vi "Run Static.vi"(7 "Tester":refnum<class "Tester.lvclass">, 8 "error in (no error)":errorcluster, 11 "Step in":refnum<class "Step.lvclass">) -> (0 "error out":errorcluster, 3 "Step out":refnum<class "Step.lvclass">)   [LabVIEW 2020, in "Tester.lvlib" / "Step.lvclass"]
uses:
  Step.lvclass
  Tester/Tester.lvclass
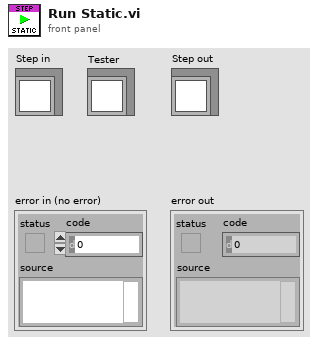
[diagram p1: front panel]
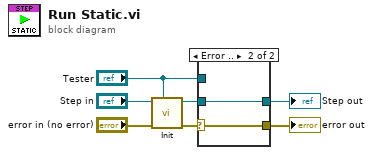
[diagram p0: block diagram]
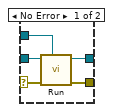
[diagram p2: hidden frame]
diagram:
  n1 = call-dynamic "Init.vi"("Tester"="Tester", "error in (no error)"="error in (no error)", "Step in"="Step in") -> ("error out"=w5:errorcluster, "Step out"=w4:refnum<class "Step.lvclass">)  [unwired: 7 in]
  n2 = case shown="Error .." w5 {
    selector: w5 -> [w11 w13]
    tunnel: w4 -> [w12 w14]
    tunnel: [w10 w14] -> w1
    tunnel: "Tester" -> [w9 _]
    tunnel: [w8 w13] -> w2
    frame No Error {
      n3 = call-dynamic "Run.vi"("Tester"=w9, "error in (no error)"=w11, "Step in"=w12) -> ("error out"=w8:errorcluster, "Step out"=w10:refnum<class "Step.lvclass">)  [unwired: 7 in]
    }
    frame Error {
    }
  }
  "error out" <- w2
  "Step out" <- w1
